vi "SpectralScan.vi"(8 "Threshold":dbl, 9 "Band Size":dbl, 10 "Start Band":dbl, 11 "Array":dbl[][](array[numeric])) -> (2 "Signal?":bool, 3 "Array 2":dbl[](array[numeric]))   [LabVIEW 2020]
panel:
  out "subarray":dbl[](array[numeric])
  out "Average":dbl
  out "element":i32
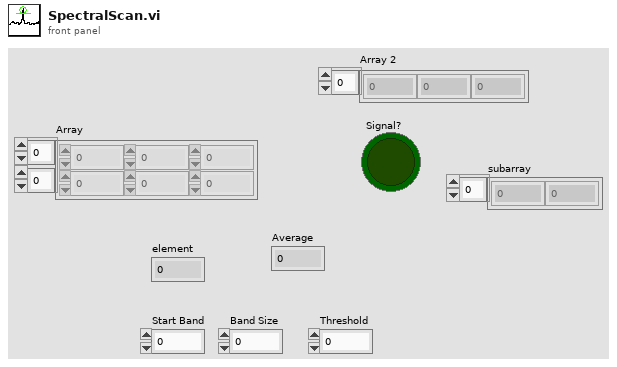
[diagram p1: front panel]
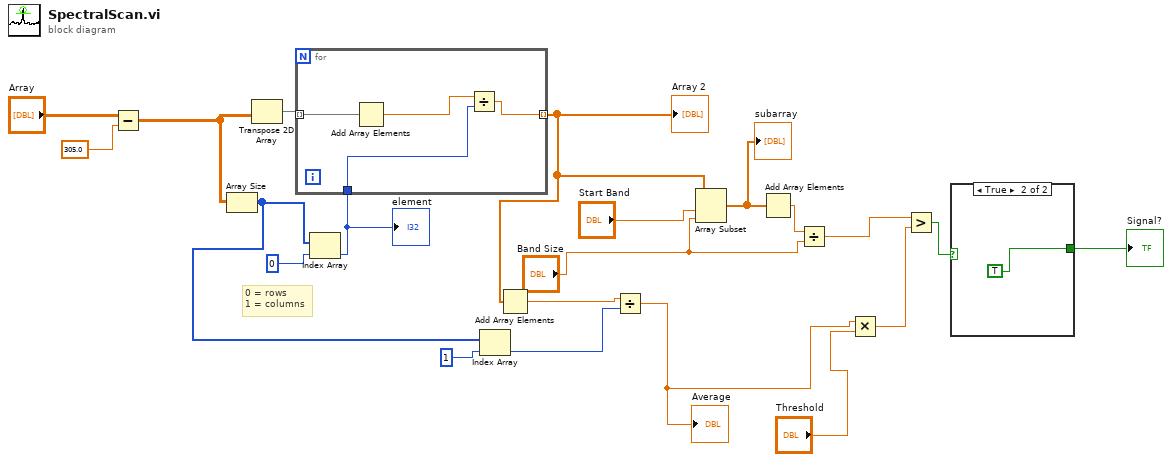
[diagram p0: block diagram]
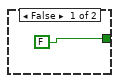
[diagram p2: hidden frame]
diagram:
  # "0 = rows \n1 = columns"
  n1 = Subtract(x="Array", y=305.0) -> (x-y=w2:dbl[][])
  n2 = Array Size(array=w2) -> (size(s)=w13:i32[])
  n3 = Transpose 2D Array(2D array=w2) -> (transposed array=w21:dbl[][])
  n4 = Index Array(array=w13, index=0) -> (element=w14:i32)
  "element" <- w14
  n5 = for {
    tunnel: w21 -> [w25] mode=indexing
    tunnel: [w23] -> w17 mode=indexing
    tunnel: w14 -> [w22]
    n6 = Add Array Elements(numeric array=w25) -> (sum=w24:dbl)
    n7 = Divide(x=w24, y=w22) -> (x/y=w23:dbl)
  }
  "Array 2" <- w17
  n8 = Index Array(array=w13, index=1) -> (element=w11:i32)
  n9 = Add Array Elements(numeric array=w17) -> (sum=w16:dbl)
  n10 = Divide(x=w16, y=w11) -> (x/y=w8:dbl)
  "Average" <- w8
  n11 = Array Subset(array=w17, index="Start Band", length="Band Size") -> (w20:dbl[])
  "subarray" <- w20
  n12 = Add Array Elements(numeric array=w20) -> (sum=w10:dbl)
  n13 = Divide(x=w10, y="Band Size") -> (x/y=w9:dbl)
  n14 = Multiply(x=w8, y="Threshold") -> (x*y=w7:dbl)
  n15 = Greater?(x=w9, y=w7) -> (0:w19:bool)
  n16 = case shown="True" w19 {
    tunnel: [FALSE TRUE] -> w18
    frame False {
    }
    frame True {
    }
  }
  "Signal?" <- w18
